vi "FormPrincipal.vi"() -> ()   [LabVIEW 2014]
uses:
  Control 1.ctl
panel:
  in  "exitButton":bool
  in  "stopButton":bool
  in  "startButton":bool
  out "Freio":bool
  out "Ensaio":bool
  out "Motor":bool
  out "String":string
  out "currentCycle 2":string
  out "currentCycle":string
  in  "freioButton":bool caption="Motor"
  in  "Cluster":T1={"ensaioButton"=FALSE, "calibraButton"=FALSE, "confGeralButton"=TRUE}
  out "ledVibracao":bool caption="Vibração"
  out "ledCarga":bool caption="Força"
  out "ledRotacao":bool caption="Rotação"
  out "ledTermoparRef":bool caption="Temp Referencia"
  out "ledTermoparB":bool caption="Temperatura 2"
  out "ledTermoparA":bool caption="Temperatura  1"
  in  "pathToFile":path
  in  "motorButton":bool caption="Motor"
  out "Enum":T2
  # "Bancada de Frenagem - Ensaio"
  # "Sensores"
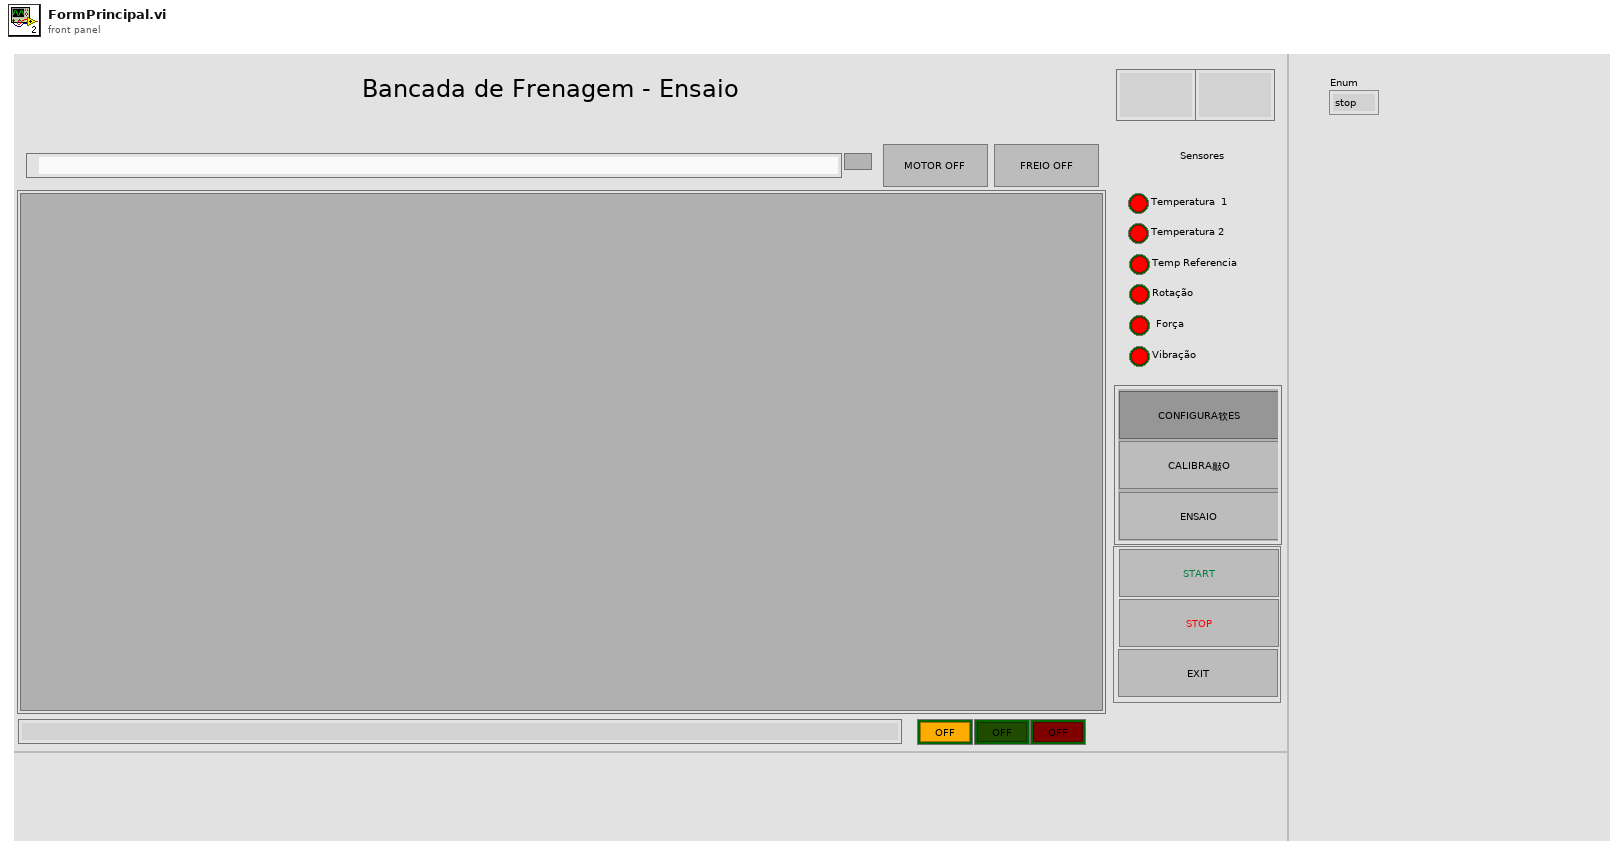
[diagram p1: front panel]
types:
  T1 = cluster{"ensaioButton":bool, "calibraButton":bool, "confGeralButton":bool}
  T2 = typedef "Control 1.ctl" = enum16{"stop", "ready", "init"}
  T3 = cluster{"confGeralButton":bool, "calibraButton":bool, "ensaioButton":bool}
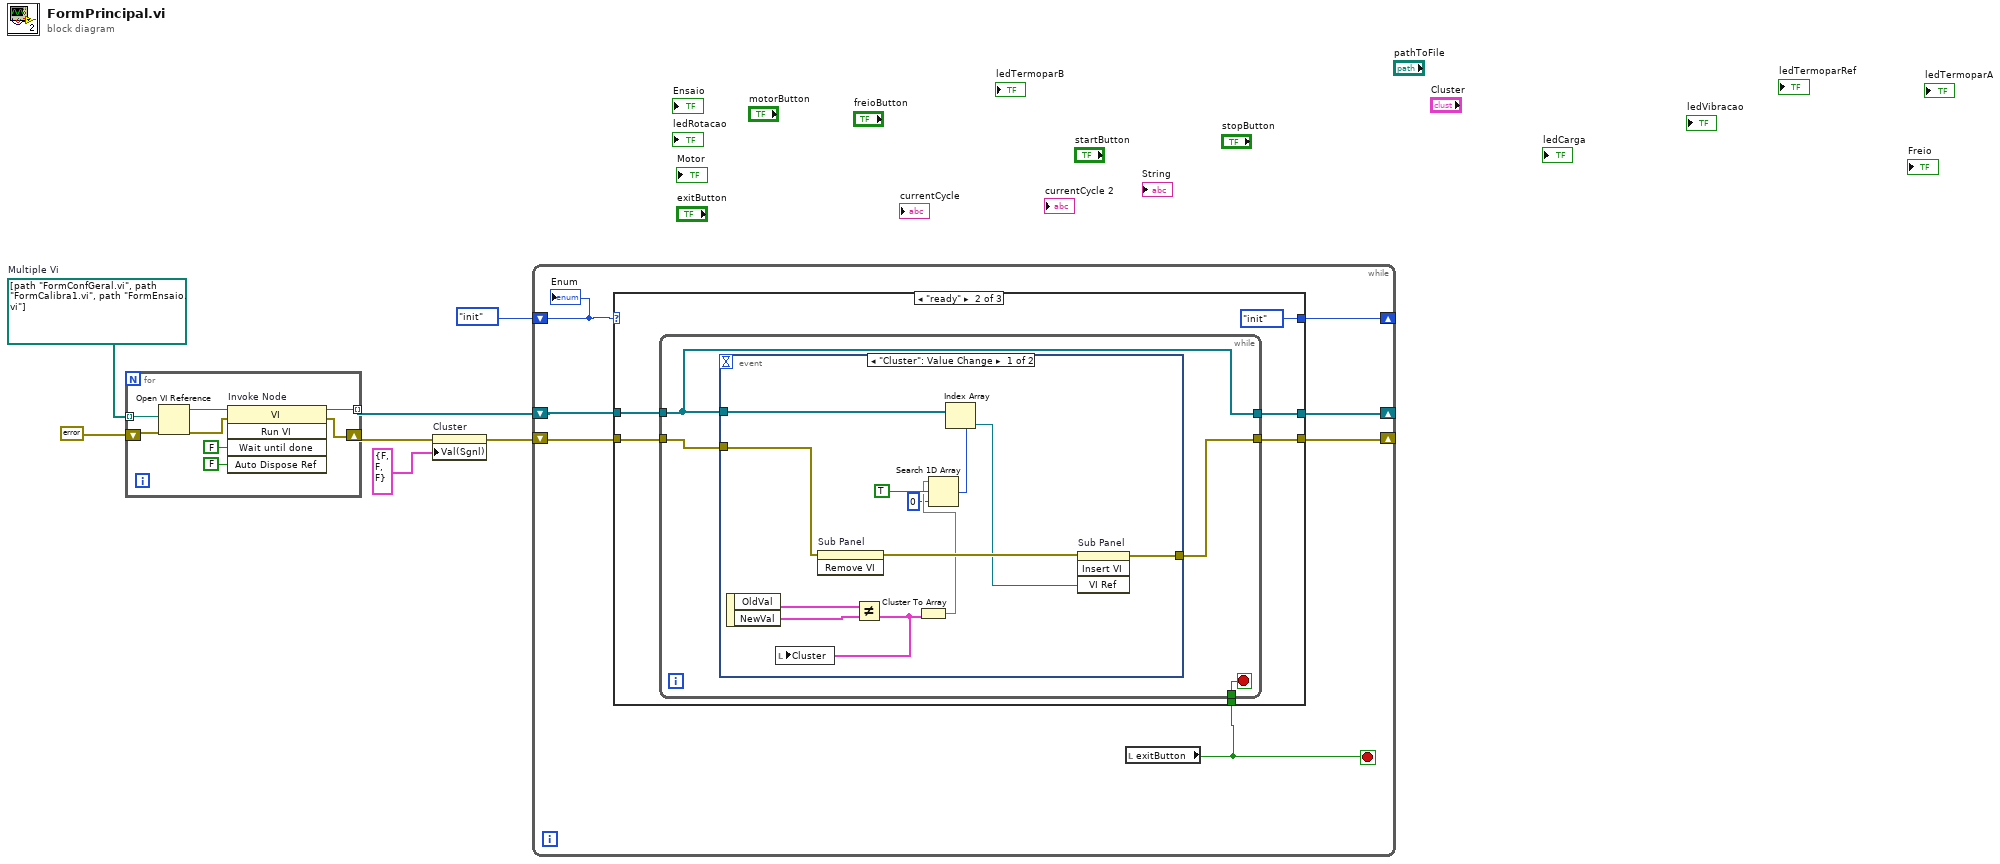
[diagram p0: block diagram]
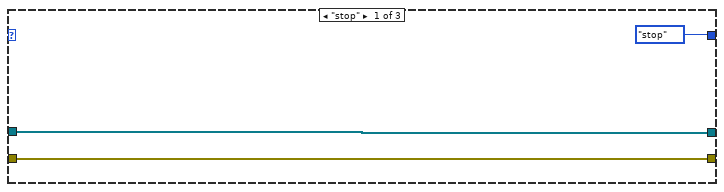
[diagram p2: hidden frame]
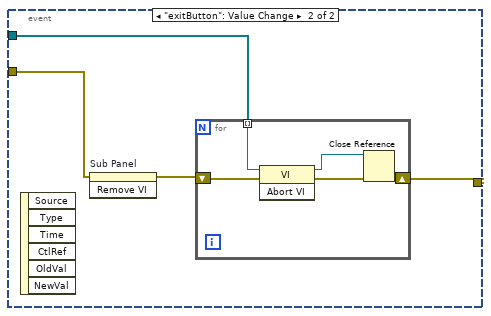
[diagram p3: hidden frame]
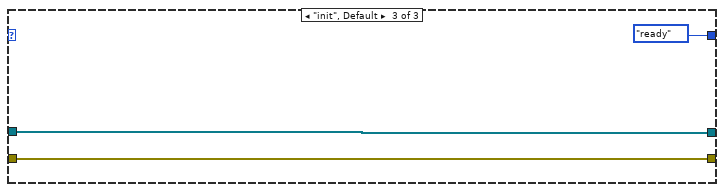
[diagram p4: hidden frame]
diagram:
  w7 = path[] [path "FormConfGeral.vi", path "FormCalibra1.vi", path "FormEnsaio.vi"]  # Multiple Vi
  n1 = for {
    tunnel: w7 -> [w15] mode=indexing
    shift-right: [w13] -> w4
    shift-left: errorcluster {FALSE, 0, ""} -> [w8]
    tunnel: [w12] -> w6 mode=indexing
    n2 = Open VI Reference(vi path=w15, error in (no error)=w8) -> (vi reference=w14:refnum<vi>, error out=w9:errorcluster)  [unwired: 4 in]
    n3 = invoke on="Invoke Node" class="VI" method="Run VI"(reference=w14, error in=w9, "Wait until done"=FALSE ("Wait Until Done"), "Auto Dispose Ref"=FALSE ("Auto Dispose Reference")) -> (reference out=w12:refnum<vi>, error out=w13:errorcluster)  [unwired: 1 in, 3 out]
  }
  n4 = property on="Cluster" class="Clust (strict)"(error in=w4, "Val(Sgnl)"=T3 {"confGeralButton"=FALSE, "calibraButton"=FALSE, "ensaioButton"=FALSE} ("Value (Signaling)")) -> (error out=w5:errorcluster)  [unwired: 1 in, 1 out]
  n5 = while {
    shift-right: [w17] -> _
    shift-left: Control_1."init" ("Enum") -> [w18]
    shift-right: [w19] -> _
    shift-left: w5 -> [w22]
    shift-right: [w20] -> _
    shift-left: w6 -> [w21]
    stop <- w16 stop-if-true
    n6 = local read "exitButton"() -> (w16:bool)
    n7 = case shown="\"ready\"" w18 {
      tunnel: w22 -> [w24 w31 w58]
      tunnel: w21 -> [w25 w30 w59]
      tunnel: [w25 w27 w59] -> w20
      tunnel: w16 -> [_ w29 _]
      tunnel: [w24 w28 w58] -> w19
      tunnel: [Control_1."stop" ("Enum") Control_1."init" ("Enum") Control_1."ready" ("Enum")] -> w17
      frame "stop" {
      }
      frame "ready" {
        n8 = while {
          tunnel: w31 -> [w35]
          tunnel: w30 -> [w32]
          tunnel: w29 -> [w34]
          tunnel: [w33] -> w28
          tunnel: [w32] -> w27
          stop <- w34 stop-if-true
          n9 = event shown="[0] \"Cluster\": Value Change" {
            selector: _ -> [_ _]
            dyn-events: _ -> [_ _]
            timeout: _ -> [_ _]
            tunnel: w32 -> [w46 w51]
            tunnel: [w45 w49] -> w33
            tunnel: w35 -> [w36 w48]
            event "Cluster": Value Change {
              n10 = event-data() -> ("OldVal"=w43:T1, "NewVal"=w42:T1)  [unwired: 1 in]
              n11 = invoke on="Sub Panel" class="SubPnl" method="Remove VI"(error in=w36) -> (error out=w47:errorcluster)  [unwired: 2 in, 2 out]
              n12 = Not Equal?(x=w43, y=w42) -> (x != y?=w39:T1)
              n13 = local write "Cluster"(w39) -> ()
              n14 = Cluster To Array(cluster=w39) -> (array=w38:bool[])
              n15 = Search 1D Array(1D array=w38, element=TRUE, start index (0)=0) -> (index of element=w41:i32)
              n16 = Index Array(array=w46, index=w41) -> (element=w44:refnum<vi>)
              n17 = invoke on="Sub Panel" class="SubPnl" method="Insert VI"(error in=w47, "VI Ref"=w44) -> (error out=w45:errorcluster)  [unwired: 2 in, 3 out]
            }
            event "exitButton": Value Change {
              n18 = event-data() -> ()  [unwired: 1 in, 6 out]
              n19 = invoke on="Sub Panel" class="SubPnl" method="Remove VI"(error in=w48) -> (error out=w50:errorcluster)  [unwired: 2 in, 2 out]
              n20 = for {
                tunnel: w51 -> [w56] mode=indexing
                shift-right: [w53] -> w49
                shift-left: w50 -> [w54]
                n21 = invoke class="VI" method="Abort VI"(reference=w56, error in=w54) -> (reference out=w52:refnum<vi>, error out=w55:errorcluster)  [unwired: 1 in, 1 out]
                n22 = Close Reference(reference=w52, error in (no error)=w55) -> (error out=w53:errorcluster)
              }
            }
          }
        }
      }
      frame "init", Default {
      }
    }
    "Enum" <- w18
  }
